vi "Write WS Message Broker Interface Ref.vi"(10 "WS Message Broker Interface Ref.lvclass":refnum<class "WS Message Broker Interface Ref.lvclass">, 11 "Controller in":refnum<class "Controller.lvclass">) -> (3 "Controller out":refnum<class "Controller.lvclass">)   [LabVIEW 2016]
uses:
  <userlib>/Common Components/Controller/Controller.lvclass
  C:/Program Files (x86)/National Instruments/LabVIEW 2016/vi.lib/ActorFramework/Actor/Actor.lvclass
  <userlib>/Common Components/WebSocket Networking/WS Message Broker Interface Ref/WS Message Broker Interface Ref.lvclass
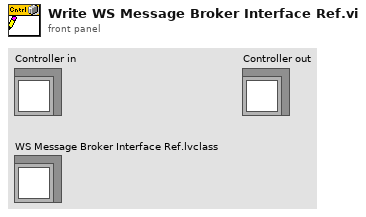
[diagram p1: front panel]
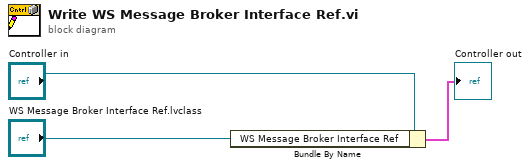
[diagram p0: block diagram]
diagram:
  n1 = Bundle By Name(cluster="Controller in", "WS Message Broker Interface Ref"="WS Message Broker Interface Ref.lvclass") -> (→"Controller out":cluster{})
